vi "handler_measurement.vi"(8 "error in (no error)":errorcluster, 10 "Server Variables":T1 {"Energy Levels"."E1" format="%_6g"; "Phases"."ExtTriggerDelay" format="%.3g"}, 11 "HTTP Request in":T7) -> (0 "error out":errorcluster, 2 "Server Variables":T1 {"Energy Levels"."E1" format="%_6g"; "Phases"."ExtTriggerDelay" format="%.3g"}, 3 "HTTP Request out":T7)   [LabVIEW 2011]
uses:
  http_request_response.ctl
  http_request.ctl
  http_field.ctl
  http_response.ctl
  template_field.ctl
  template_field_type.ctl
  Server Variables.ctl
  Phase Parameters.ctl
  Phase Mode.ctl
  Energy Level_.ctl
  Measurement Parameters.ctl
  Results.ctl
  JSON BDP Result.ctl
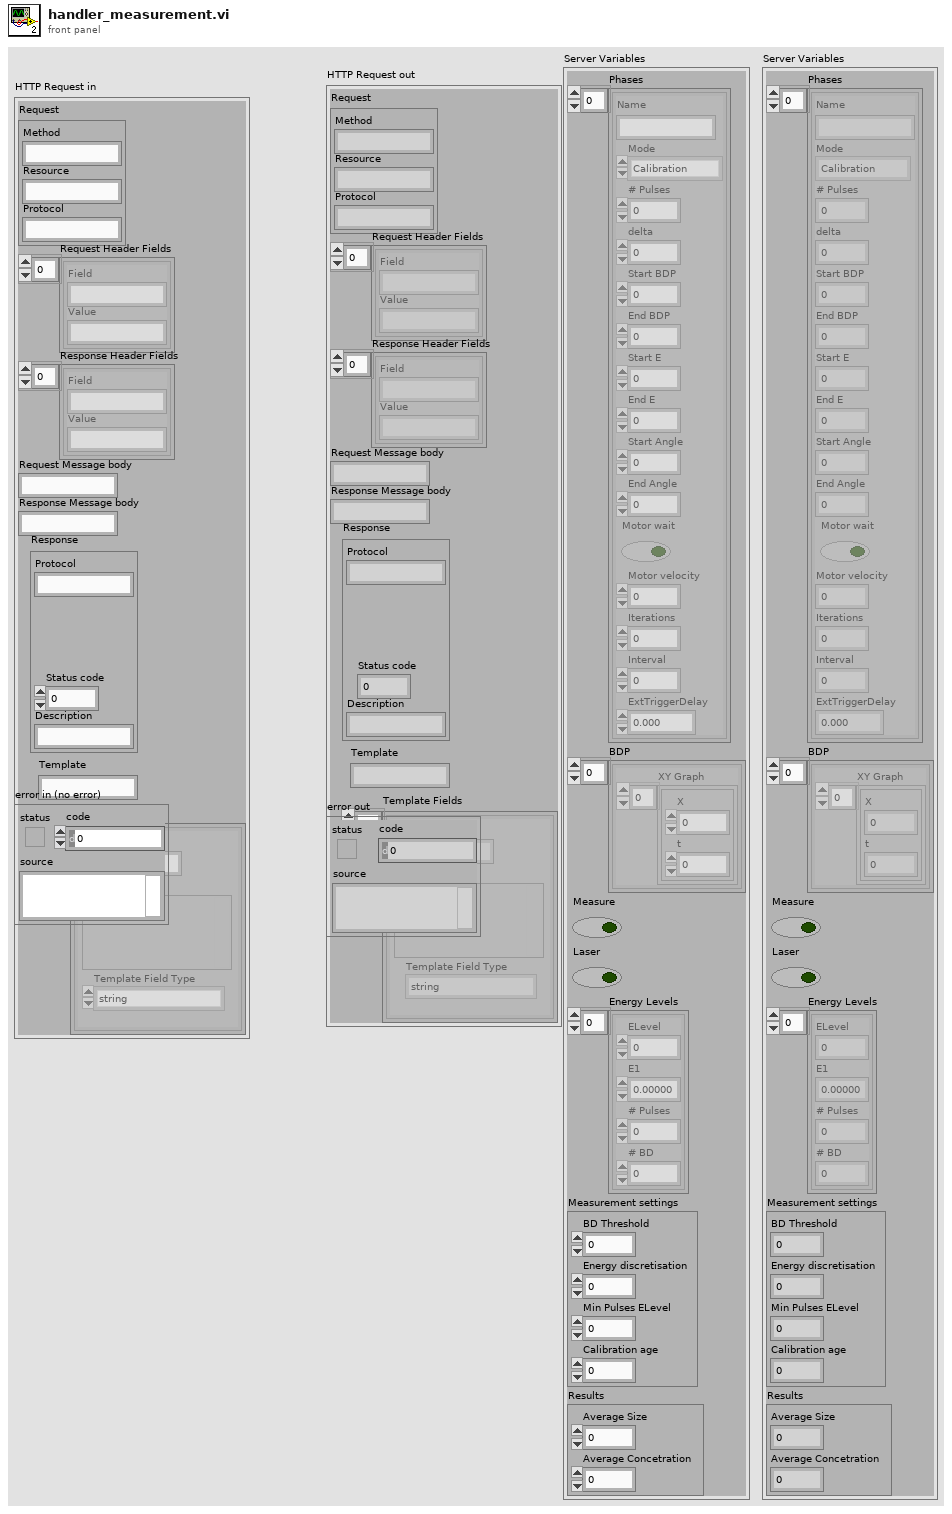
[diagram p1: front panel]
types:
  T1 = typedef "Server Variables.ctl" = cluster{"Phases":T2[], "BDP":cluster{"XY Graph":cluster{"X":dbl, "t":dbl}[]}[], "Measure":bool, "Laser":bool, "Energy Levels":T4[], "Measurement settings":T5, "Results":T6}
  T2 = typedef "Phase Parameters.ctl" = cluster{"Name":string, "Mode":T3, "# Pulses":u32, "delta":dbl, "Start BDP":dbl, "End BDP":dbl, "Start E":dbl, "End E":dbl, "Start Angle":dbl, "End Angle":dbl, "Motor wait":bool, "Motor velocity":dbl, "Iterations":dbl, "Interval":dbl, "ExtTriggerDelay":dbl}
  T3 = typedef "Phase Mode.ctl" = enum16{"Calibration", "Linear", "BDP-Fit", "Raw"}
  T4 = typedef "Energy Level_.ctl" = cluster{"ELevel":dbl, "E1":dbl, "# Pulses":i32, "# BD":i32}
  T5 = typedef "Measurement Parameters.ctl" = cluster{"BD Threshold":dbl, "Energy discretisation":i32, "Min Pulses ELevel":i32, "Calibration age":i32}
  T6 = typedef "Results.ctl" = cluster{"Average Size":dbl, "Average Concetration":dbl}
  T7 = typedef "http_request_response.ctl" = cluster{"Request":T8, "Request Header Fields":T9[], "Response Header Fields":T9[], "Request Message body":string, "Response Message body":string, "Response":T10, "Template":string, "Template Fields":T11[]}
  T8 = typedef "http_request.ctl" = cluster{"Method":string, "Resource":string, "Protocol":string}
  T9 = typedef "http_field.ctl" = cluster{"Field":string, "Value":string}
  T10 = typedef "http_response.ctl" = cluster{"Protocol":string, "Status code":dbl, "Description":string}
  T11 = typedef "template_field.ctl" = cluster{"Name":string, "Template Field Type":T12, "data":variant}
  T12 = typedef "template_field_type.ctl" = enum16{"string", "string array", "number", "number array", "cluster", "cluster array"}
  T13 = typedef "JSON BDP Result.ctl" = cluster{"bdp":cluster{"E":dbl, "BDP":dbl}[], "diameter":dbl, "concentration":dbl}
  T14 = cluster{"XY Graph":cluster{"X":dbl, "t":dbl}[]}[]
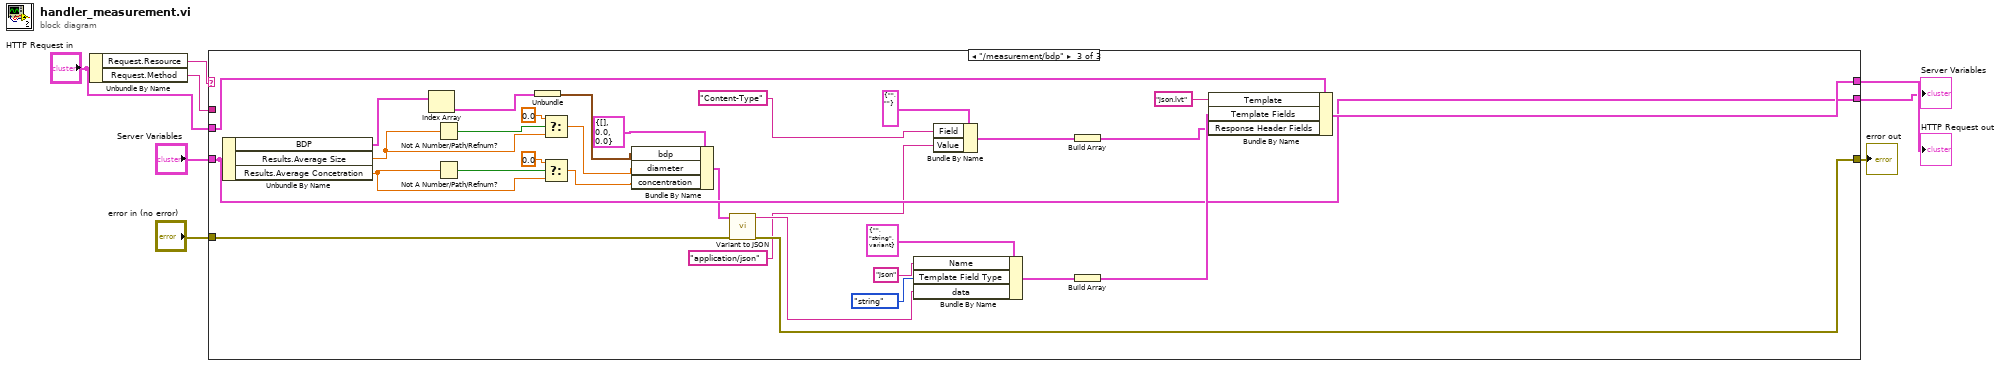
[diagram p0: block diagram]
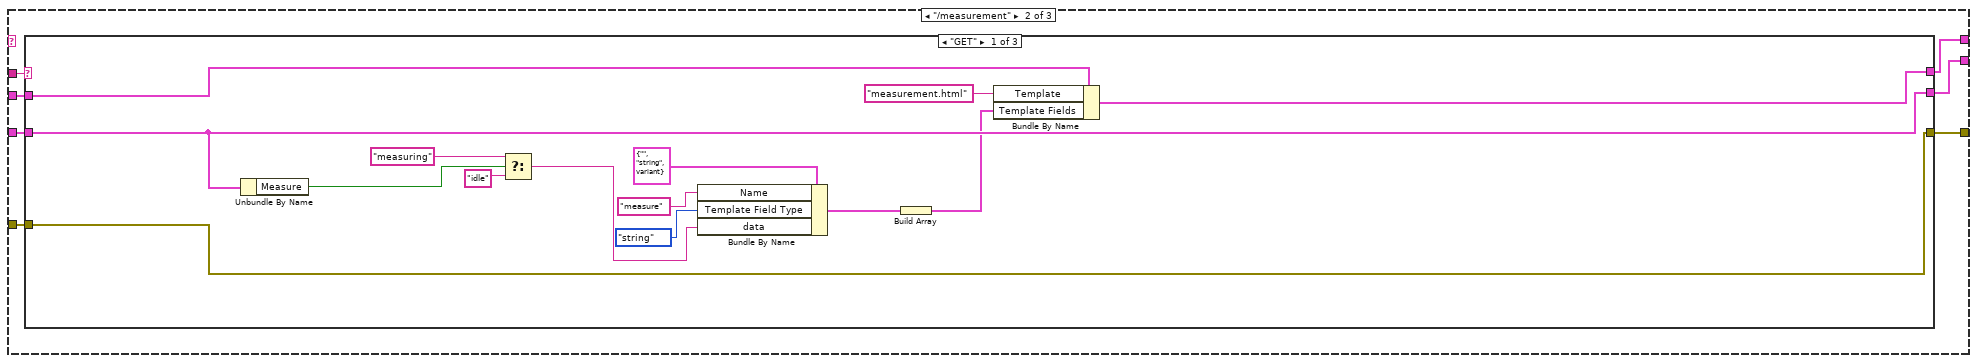
[diagram p3: hidden frame]
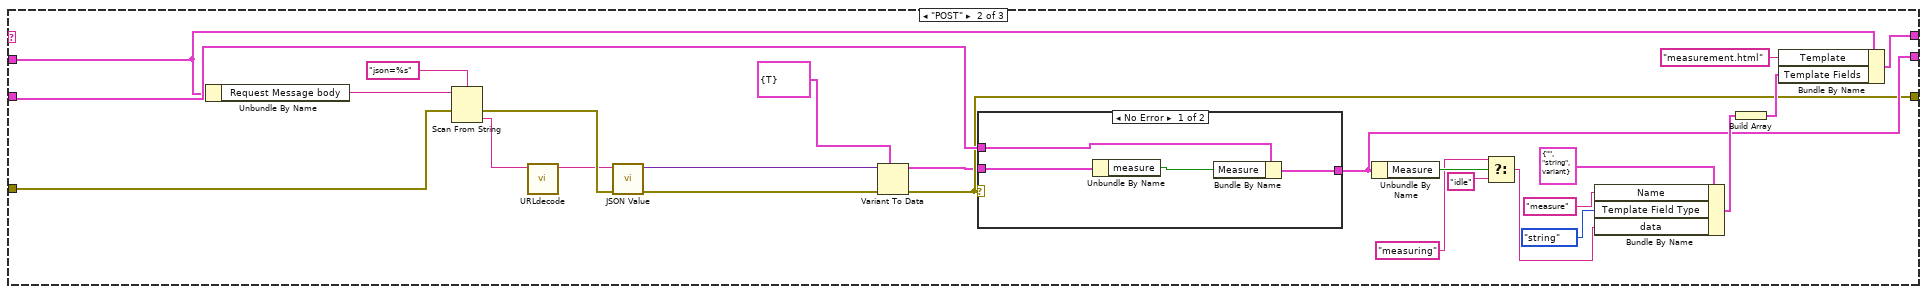
[diagram p4: hidden frame]
diagram:
  n1 = Unbundle By Name("HTTP Request in") -> ("Request.Resource"=w8:string, "Request.Method"=w7:string)
  n2 = case shown="\"/measurement/bdp\"" w8 {
    tunnel: w7 -> [_ w18 _]
    tunnel: "HTTP Request in" -> [w11 w17 w94]
    tunnel: [w11 w16 w95] -> w5
    tunnel: "error in (no error)" -> [w10 w15 w83]
    tunnel: [w10 w14 w82] -> w3
    tunnel: "Server Variables" -> [w9 w13 w86]
    tunnel: [w9 w12 w86] -> w1
    frame Default {
    }
    frame "/measurement" {
      n3 = case shown="\"GET\"" w18 {
        tunnel: w17 -> [w30 w45 w65]
        tunnel: [w32 w57 w65] -> w16
        tunnel: w15 -> [w27 w42 w64]
        tunnel: [w27 w37 w64] -> w14
        tunnel: w13 -> [w29 w46 w63]
        tunnel: [w29 w44 w63] -> w12
        frame "GET" {
          n4 = Unbundle By Name(w29) -> ("Measure"=w22:bool)
          n5 = Select(t="measuring", s=w22, f="idle") -> (s? t:f=w19:string)
          n6 = Bundle By Name(cluster=T11 {"Name"="", "Template Field Type"=enum."string", "data"=variant} ("Template Field"), "Name"="measure", "Template Field Type"=template_field_type."string", "data"=w19) -> (w25:T11)
          n7 = Build Array(w25) -> (w28:T11[])
          n8 = Bundle By Name(cluster=w30, "Template"="measurement.html", "Template Fields"=w28) -> (w32:T7)
        }
        frame "POST" {
          n9 = Unbundle By Name(w45) -> ("Request Message body"=w43:string)
          n10 = Scan From String(format string="json=%s", input string=w43, error in=w42) -> (error out=w38:errorcluster, output 1=w34:string)  [unwired: 2 in, 2 out]
          n11 = call "URLdecode.vi"("URL encoded in"=w34) -> ("URL encoded out"=w33:string)  [unwired: 10 in]
          n12 = call "JSON Value.vi"("error in (no error)"=w38, "JSON"=w33) -> ("error out"=w40:errorcluster, "Value"=w39:variant)  [unwired: 7 in, 1 out]
          n13 = Variant To Data(error in=w40, type=cluster{"measure":bool} {"measure"=TRUE}, Variant=w39) -> (data=w36:cluster{"measure":bool}, error out=w37:errorcluster)
          n14 = case shown="No Error" w37 {
            tunnel: w46 -> [w61 w62]
            tunnel: [w60 w62] -> w44
            tunnel: w36 -> [w59 _]
            frame No Error {
              n15 = Unbundle By Name(w59) -> ("measure"=w58:bool)
              n16 = Bundle By Name(cluster=w61, "Measure"=w58) -> (w60:T1)
            }
            frame Error {
            }
          }
          n17 = Unbundle By Name(w44) -> ("Measure"=w51:bool)
          n18 = Select(t="measuring", s=w51, f="idle") -> (s? t:f=w48:string)
          n19 = Bundle By Name(cluster=T11 {"Name"="", "Template Field Type"=enum."string", "data"=variant} ("Template Field"), "Name"="measure", "Template Field Type"=template_field_type."string", "data"=w48) -> (w54:T11)
          n20 = Build Array(w54) -> (w47:T11[])
          n21 = Bundle By Name(cluster=w45, "Template"="measurement.html", "Template Fields"=w47) -> (w57:T7)
        }
        frame Default {
        }
      }
    }
    frame "/measurement/bdp" {
      n22 = Unbundle By Name(w86) -> ("BDP"=w85:T14, "Results.Average Size"=w67:dbl, "Results.Average Concetration"=w69:dbl)
      n23 = Index Array(array=w85) -> (element=w84:cluster{"XY Graph":cluster{"X":dbl, "t":dbl}[]})  [unwired: 1 in]
      n24 = Not A Number/Path/Refnum?(number/path/refnum=w67) -> (NaN/Path/Refnum?=w72:bool)
      n25 = Not A Number/Path/Refnum?(number/path/refnum=w69) -> (NaN/Path/Refnum?=w73:bool)
      n26 = Unbundle(w84) -> ("XY Graph"=w75:cluster{"X":dbl, "t":dbl}[])
      n27 = Select(t=0.0, s=w72, f=w67) -> (s? t:f=w66:dbl)
      n28 = Select(t=0.0, s=w73, f=w69) -> (s? t:f=w68:dbl)
      n29 = Bundle By Name(cluster=T13 {"bdp"=[], "diameter"=0.0, "concentration"=0.0}, "bdp"=w75, "diameter"=w66, "concentration"=w68) -> (w74:T13)
      n30 = call "Variant to JSON.vi"("error in"=w83, "variant"=w74) -> ("error out"=w82:errorcluster, "concatenated string"=w87:string)  [unwired: 8 in]
      n31 = Bundle By Name(cluster=T11 {"Name"="", "Template Field Type"=enum."string", "data"=variant} ("Template Field"), "Name"="json", "Template Field Type"=template_field_type."string", "data"=w87) -> (w92:T11)
      n32 = Bundle By Name(cluster=T9 {"Field"="", "Value"=""} ("Header Field"), "Field"="Content-Type", "Value"="application/json") -> (w79:T9)
      n33 = Build Array(w79) -> (w81:T9[])
      n34 = Build Array(w92) -> (w91:T11[])
      n35 = Bundle By Name(cluster=w94, "Template"="json.lvt", "Template Fields"=w91, "Response Header Fields"=w81) -> (w95:T7)
    }
  }
  "HTTP Request out" <- w5
  "error out" <- w3
  "Server Variables" <- w1
